vi "UI Initialize.vi"(8 "error in (no error)":errorcluster, 11 "UI ActorTop in":refnum<class "UI_Top_Customer.lvclass">) -> (0 "error out":errorcluster, 3 "UI ActorTop out":refnum<class "UI_Top_Customer.lvclass">)   [LabVIEW 2021, in "UI_Top_Customer.lvclass"]
doc: "UI: Initialize\n2015-03-18 16:27:22\n蒋松\njiangsong@outlook.com"
uses:
  UI_Top_Customer.lvclass
  UI_Top_Customer.lvclass/UI_Top_Customer.ctl
  <userlib>/John_Lib/AbstractActorTemplate/AbstractActorTemplate/UIActorTop.lvclass
  <userlib>/John_Lib/TopPath/TopPath.lvlib
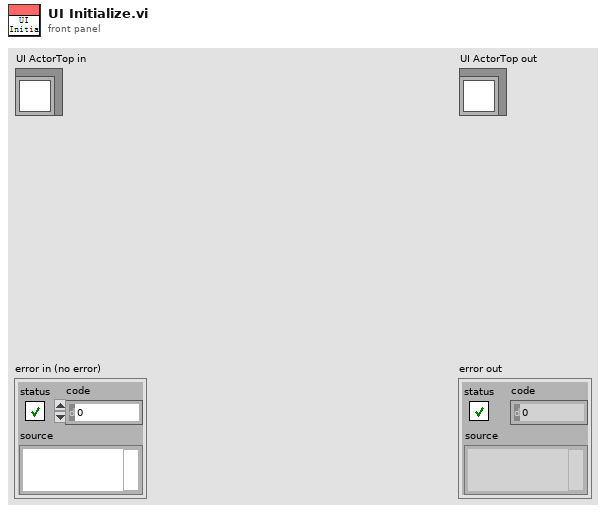
[diagram p1: front panel]
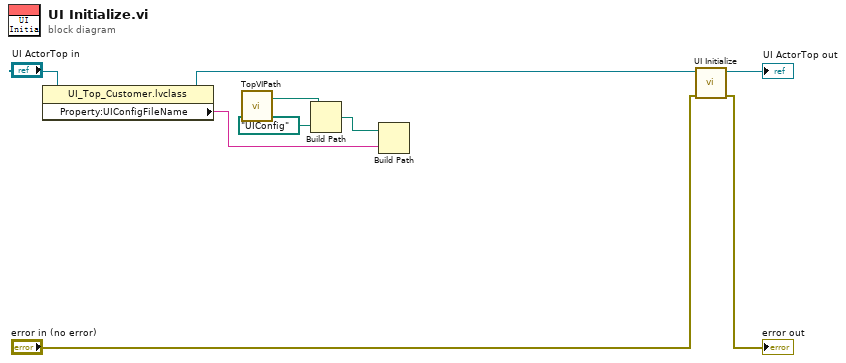
[diagram p0: block diagram]
diagram:
  n1 = property class="UI_Top_Customer.lvclass"(reference="UI ActorTop in") -> (reference out=w2:refnum<class "UI_Top_Customer.lvclass">, "Property:UIConfigFileName"=w6:string)  [unwired: 1 in, 1 out]
  n2 = call <userlib>:"TopVIPath.vi"() -> ("ConfigFile path"=w1:path)  [unwired: 1 in, 2 out]
  n3 = Build Path(base path=w1, name or relative path=path "UIConfig") -> (appended path=w5:path)
  n4 = Build Path(base path=w5, name or relative path=w6) -> ()  [unwired: 1 out]
  n5 = call-parent "UI Initialize.vi"("error in (no error)"="error in (no error)", "UI ActorTop in"=w2) -> ("error out"=→"error out":errorcluster, "UI ActorTop out"=→"UI ActorTop out":refnum<class "UI_Top_Customer.lvclass">)  [unwired: 8 in]
